vi "FTW-Event-FlattenJSON.vi"(0 "Event JSON String":string, 2 "UTC":bool, 11 "error in":errorcluster) -> (4 "Flattened Event":string, 15 "error out":errorcluster)   [LabVIEW 2013]
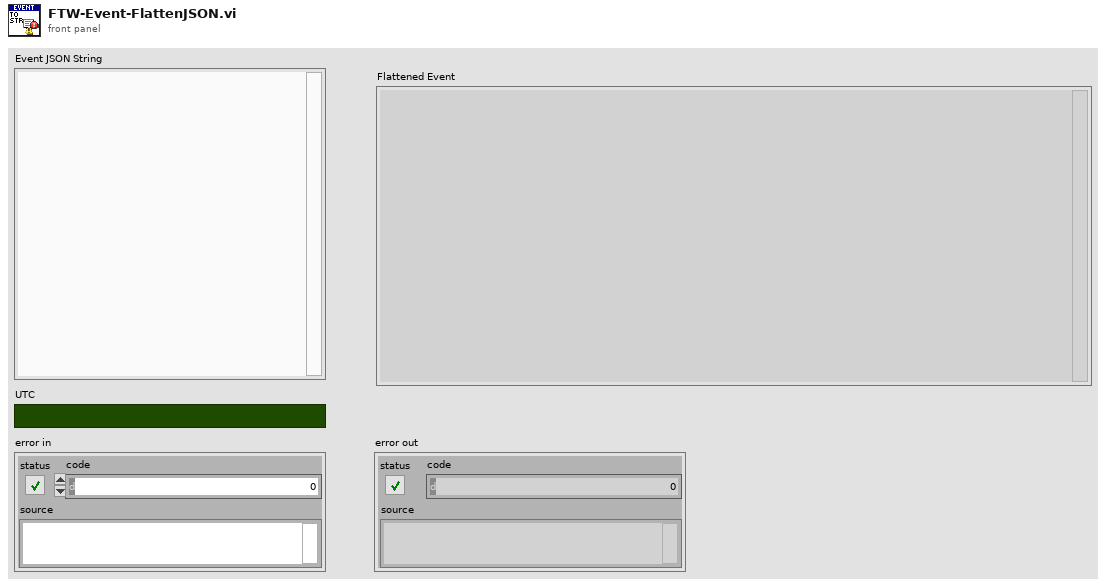
[diagram p1: front panel]
types:
  T1 = typedef "FTW-Event.ctl" = cluster{"Count":i32, "Uptime":dbl, "Timestamp":timestamp, "Source":string, "Type":string, "Data":string, "Error":errorcluster}
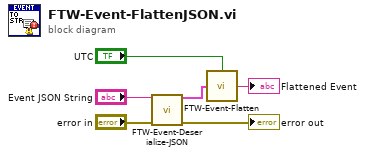
[diagram p0: block diagram]
diagram:
  n1 = call "FTW-Event-Deserialize-JSON.vi"("Serialized Event"="Event JSON String", "error in"="error in") -> ("Event"=w3:T1, "error out"=→"error out":errorcluster)  [unwired: 12 in]
  n2 = call "FTW-Event-Flatten.vi"("UTC"="UTC", "Event"=w3) -> ("Flattened Event"=→"Flattened Event":string)  [unwired: 13 in]
